vi "Master_DAQ_convertUnits.vi"(1 "Raw data in":T1={"cRIO Data"={"Time (ms)"=0.0, "24V Battery (V)"=0.0, "LowV Current (A)"=0.0, "Fiducial Sensor (V)"=0.0, "PV Pressure (psig)"=0.0, "Flow Sensor (V)"=0.0, "Temp Fairing (F)"=0.0, "Temp Reservoir (F)"=0.0, "HallEffect Right (in)"=0.0, "HallEffect Left (in)"=0.0, "PT Tank (psig)"=0.0, "PT Clamp Right (psig)"=0.0, "PT Clamp Left (psig)"=0.0, "PT Brake (psig)"=0.0, "PT Cooling (psig)"=0.0, "Displacement (ft)"=0.0, "Velocity (ft/s)"=0.0}, "IMU Data"={"x acceleration (g)"=0.0, "Pressure (psia)"=0.0, "Temperature (F)"=0.0}, "BMS Data"={"Max Cell Voltage (V)"=0.0, "Max Cell ID"=0.0, "Min Cell Voltage (V)"=0.0, "Min Cell ID"=0.0, "State of Charge (%)"=0.0, "Average Voltage (V)"=0.0, "Voltage Delta (V)"=0.0, "Pack Current (A)"=0.0, "Pack Voltage (V)"=0.0, "Max Resistance (Ohm)"=0.0, "Min Resistance (Ohm)"=0.0, "Average Resistance (Ohm)"=0.0, "Delta Resistance (Ohm)"=0.0, "Highest Temperature(F)"=0.0, "BmsStatus"={"isFault"=FALSE, "isolationMonitoring"=FALSE}}, "Motor Data"={"Velo (RPM)"=0.0, "MotorTemp(F)"=0.0, "CtrlTemp(F)"=0.0, "DcLinkVolt(V)"=0.0, "ErrorCode"=0.0, "motorStatus"={"isReady"=FALSE, "isOn"=FALSE, "isOperEn"=FALSE, "isFault"=FALSE, "isVoltEn"=FALSE, "targetReached"=FALSE, "isWarning"=FALSE}, "isAlive"=FALSE, "motorControllerState"=1}} {"Motor Data"."motorControllerState" items=["unknown"=1, "boot-up"=0, "stopped"=4, "operational"=5, "pre-operational"=127, "connection lost"=128]}) -> (0 "Data out":T1={"cRIO Data"={"Time (ms)"=0.0, "24V Battery (V)"=0.0, "LowV Current (A)"=0.0, "Fiducial Sensor (V)"=0.0, "PV Pressure (psig)"=0.0, "Flow Sensor (V)"=0.0, "Temp Fairing (F)"=0.0, "Temp Reservoir (F)"=0.0, "HallEffect Right (in)"=0.0, "HallEffect Left (in)"=0.0, "PT Tank (psig)"=0.0, "PT Clamp Right (psig)"=0.0, "PT Clamp Left (psig)"=0.0, "PT Brake (psig)"=0.0, "PT Cooling (psig)"=0.0, "Displacement (ft)"=0.0, "Velocity (ft/s)"=0.0}, "IMU Data"={"x acceleration (g)"=0.0, "Pressure (psia)"=0.0, "Temperature (F)"=0.0}, "BMS Data"={"Max Cell Voltage (V)"=0.0, "Max Cell ID"=0.0, "Min Cell Voltage (V)"=0.0, "Min Cell ID"=0.0, "State of Charge (%)"=0.0, "Average Voltage (V)"=0.0, "Voltage Delta (V)"=0.0, "Pack Current (A)"=0.0, "Pack Voltage (V)"=0.0, "Max Resistance (Ohm)"=0.0, "Min Resistance (Ohm)"=0.0, "Average Resistance (Ohm)"=0.0, "Delta Resistance (Ohm)"=0.0, "Highest Temperature(F)"=0.0, "BmsStatus"={"isFault"=FALSE, "isolationMonitoring"=FALSE}}, "Motor Data"={"Velo (RPM)"=0.0, "MotorTemp(F)"=0.0, "CtrlTemp(F)"=0.0, "DcLinkVolt(V)"=0.0, "ErrorCode"=0.0, "motorStatus"={"isReady"=FALSE, "isOn"=FALSE, "isOperEn"=FALSE, "isFault"=FALSE, "isVoltEn"=FALSE, "targetReached"=FALSE, "isWarning"=FALSE}, "isAlive"=FALSE, "motorControllerState"=1}} {"Motor Data"."motorControllerState" items=["unknown"=1, "boot-up"=0, "stopped"=4, "operational"=5, "pre-operational"=127, "connection lost"=128]})   [LabVIEW 2017]
uses:
  Master_DataControl.ctl
  TypeDef_cRIOData.ctl
  IMU/TypeDef_IMUData.ctl
  CAN/TypeDef_BMSData.ctl
  CAN/TypeDef_BMS_Status.ctl
  CAN/MotorController/fixedMotorData.ctl
  CAN/MotorController/MotorStatus.ctl
  CAN/MotorController/MotorData.ctl
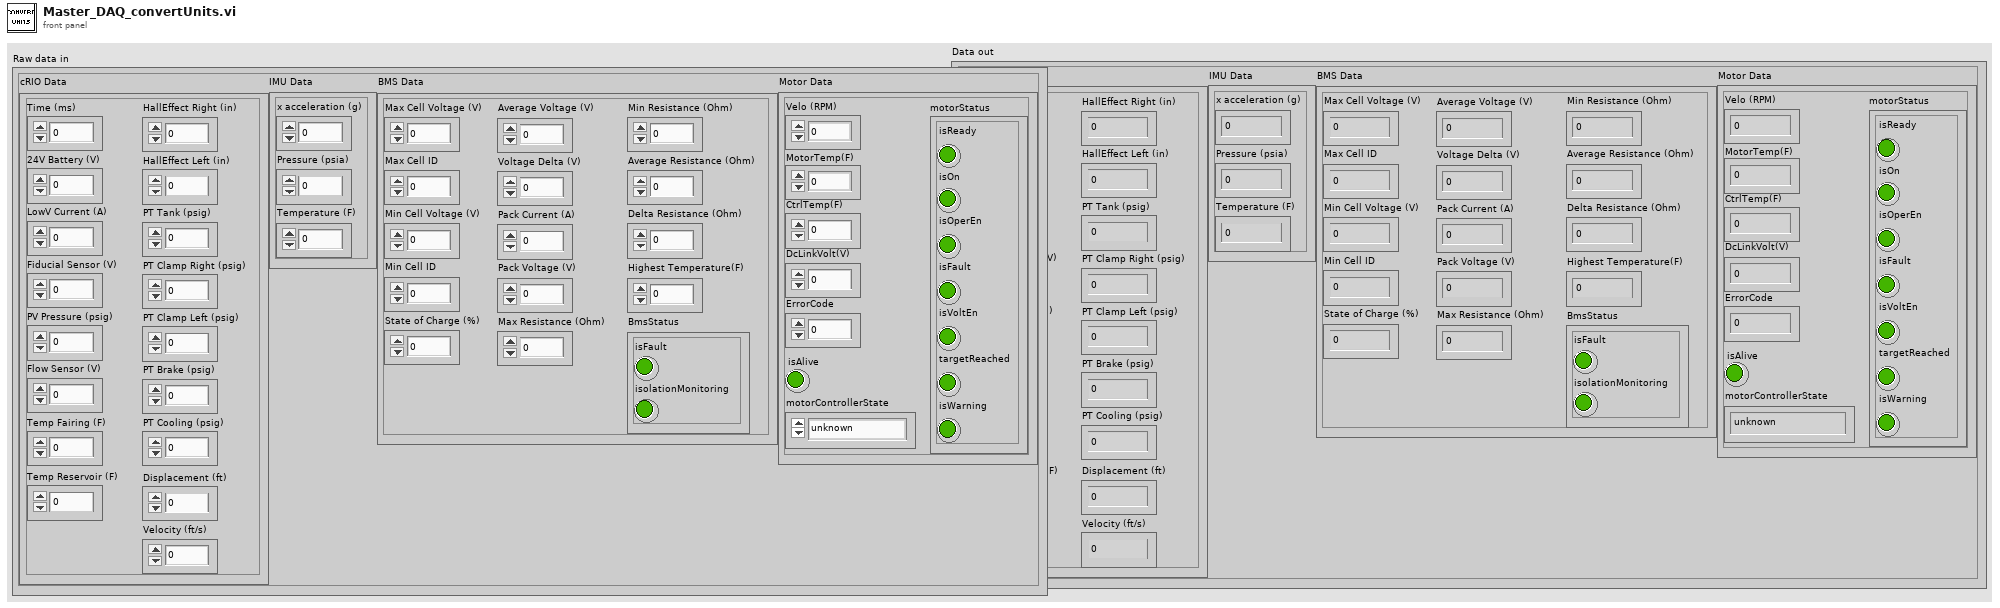
[diagram p1: front panel]
types:
  T1 = typedef "Master_DataControl.ctl" = cluster{"cRIO Data":T2, "IMU Data":T3, "BMS Data":T4, "Motor Data":T6}
  T2 = typedef "TypeDef_cRIOData.ctl" = cluster{"Time (ms)":dbl, "24V Battery (V)":dbl, "LowV Current (A)":dbl, "Fiducial Sensor (V)":dbl, "PV Pressure (psig)":dbl, "Flow Sensor (V)":dbl, "Temp Fairing (F)":dbl, "Temp Reservoir (F)":dbl, "HallEffect Right (in)":dbl, "HallEffect Left (in)":dbl, "PT Tank (psig)":dbl, "PT Clamp Right (psig)":dbl, "PT Clamp Left (psig)":dbl, "PT Brake (psig)":dbl, "PT Cooling (psig)":dbl, "Displacement (ft)":dbl, "Velocity (ft/s)":dbl}
  T3 = typedef "TypeDef_IMUData.ctl" = cluster{"x acceleration (g)":dbl, "Pressure (psia)":dbl, "Temperature (F)":dbl}
  T4 = typedef "TypeDef_BMSData.ctl" = cluster{"Max Cell Voltage (V)":dbl, "Max Cell ID":dbl, "Min Cell Voltage (V)":dbl, "Min Cell ID":dbl, "State of Charge (%)":dbl, "Average Voltage (V)":dbl, "Voltage Delta (V)":dbl, "Pack Current (A)":dbl, "Pack Voltage (V)":dbl, "Max Resistance (Ohm)":dbl, "Min Resistance (Ohm)":dbl, "Average Resistance (Ohm)":dbl, "Delta Resistance (Ohm)":dbl, "Highest Temperature(F)":dbl, "BmsStatus":T5}
  T5 = typedef "TypeDef_BMS_Status.ctl" = cluster{"isFault":bool, "isolationMonitoring":bool}
  T6 = typedef "fixedMotorData.ctl" = cluster{"Velo (RPM)":dbl, "MotorTemp(F)":dbl, "CtrlTemp(F)":dbl, "DcLinkVolt(V)":dbl, "ErrorCode":dbl, "motorStatus":T7, "isAlive":bool, "motorControllerState":u16}
  T7 = typedef "MotorStatus.ctl" = cluster{"isReady":bool, "isOn":bool, "isOperEn":bool, "isFault":bool, "isVoltEn":bool, "targetReached":bool, "isWarning":bool}
  T8 = typedef "MotorData.ctl" = cluster{"Velo (RPM)":i32, "MotorTemp(C)":u8, "CtrlTemp(C)":u8, "DcLinkVolt(V)":dbl, "ErrorCode":dbl, "isAlive":bool, "motorControllerState":u16, "motorStatus":T7}
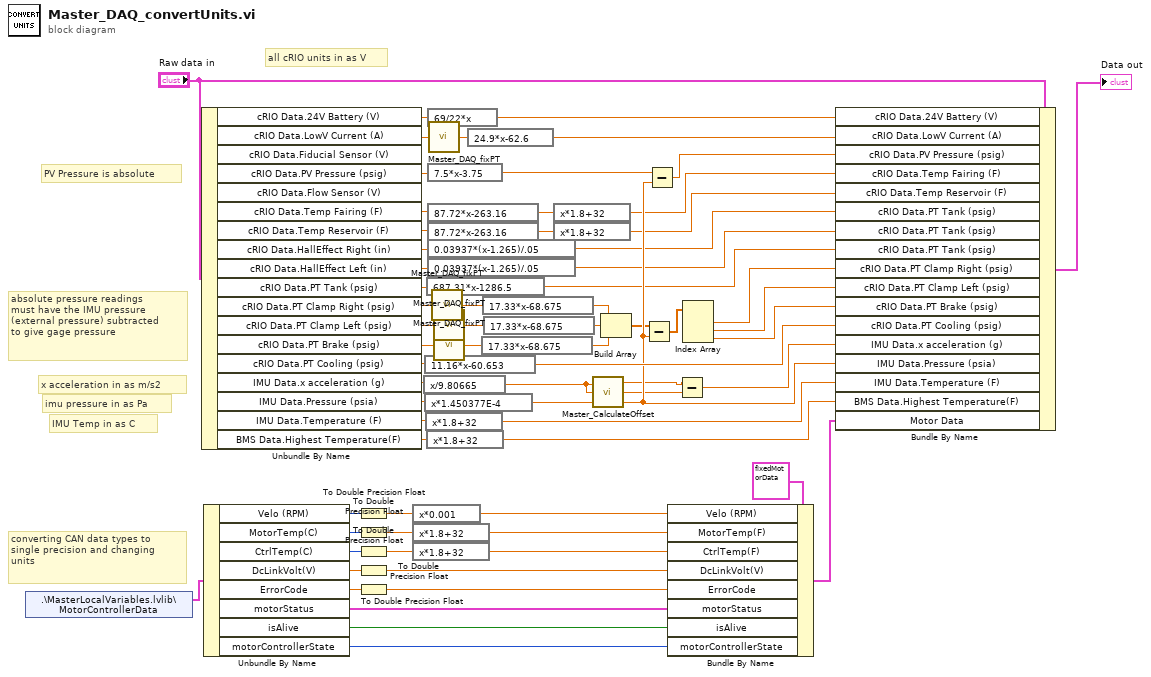
[diagram p0: block diagram]
diagram:
  # "converting CAN data types to\nsingle precision and changing\nunits"
  # "absolute pressure readings\nmust have the IMU pressure\n(external pressure) subtracted\nto give gage pressure"
  # "PV Pressure is absolute"
  # "IMU Temp in as C"
  # "imu pressure in as Pa"
  # "x acceleration in as m/s2"
  # "all cRIO units in as V"
  n1 = shared-variable ".\\MasterLocalVariables.lvlib\\MotorControllerData"() -> (w38:T8)  [unwired: 1 in, 1 out]
  n2 = Unbundle By Name("Raw data in") -> ("cRIO Data.24V Battery (V)"=w65:dbl, "cRIO Data.LowV Current (A)"=w3:dbl, "cRIO Data.PV Pressure (psig)"=w64:dbl, "cRIO Data.Temp Fairing (F)"=w63:dbl, "cRIO Data.Temp Reservoir (F)"=w62:dbl, "cRIO Data.HallEffect Right (in)"=w17:dbl, "cRIO Data.HallEffect Left (in)"=w16:dbl, "cRIO Data.PT Tank (psig)"=w61:dbl, "cRIO Data.PT Clamp Right (psig)"=w12:dbl, "cRIO Data.PT Clamp Left (psig)"=w11:dbl, "cRIO Data.PT Brake (psig)"=w10:dbl, "cRIO Data.PT Cooling (psig)"=w60:dbl, "IMU Data.x acceleration (g)"=w59:dbl, "IMU Data.Pressure (psia)"=w58:dbl, "IMU Data.Temperature (F)"=w57:dbl, "BMS Data.Highest Temperature(F)"=w56:dbl)  [unwired: 2 out]
  n3 = Unbundle By Name(w38) -> ("Velo (RPM)"=w37:i32, "MotorTemp(C)"=w35:u8, "CtrlTemp(C)"=w34:u8, "DcLinkVolt(V)"=w33:dbl, "ErrorCode"=w32:dbl, "motorStatus"=w30:T7, "isAlive"=w31:bool, "motorControllerState"=w20:u16)
  n4 = To Double Precision Float(number=w37) -> (double precision float=w29:dbl)
  n5 = To Double Precision Float(number=w35) -> (double precision float=w23:dbl)
  n6 = To Double Precision Float(number=w34) -> (double precision float=w27:dbl)
  n7 = To Double Precision Float(number=w33) -> (double precision float=w25:dbl)
  n8 = To Double Precision Float(number=w32) -> (double precision float=w26:dbl)
  n9 = expression code="x*0.001"(w29) -> (w28:dbl)
  n10 = expression code="x*1.8+32"(w23) -> (w22:dbl)
  n11 = expression code="x*1.8+32"(w27) -> (w24:dbl)
  n12 = expression code="x/9.80665"(w59) -> (w41:dbl)
  n13 = expression code="11.16*x-60.653"(w60) -> (w52:dbl)
  n14 = expression code="x*1.450377E-4"(w58) -> (w46:dbl)
  n15 = expression code="x*1.8+32"(w57) -> (w53:dbl)
  n16 = expression code="687.31*x-1286.5"(w61) -> (w15:dbl)
  n17 = expression code="x*1.8+32"(w56) -> (w54:dbl)
  n18 = expression code="69/22*x"(w65) -> (w55:dbl)
  n19 = expression code="7.5*x-3.75"(w64) -> (w48:dbl)
  n20 = expression code="87.72*x-263.16"(w63) -> (w44:dbl)
  n21 = expression code="87.72*x-263.16"(w62) -> (w45:dbl)
  n22 = expression code="0.03937*(x-1.265)/.05"(w17) -> (w13:dbl)
  n23 = expression code="0.03937*(x-1.265)/.05"(w16) -> (w14:dbl)
  n24 = call "Master_DAQ_fixPT.vi"("new value"=w3) -> ("mean"=w2:dbl)
  n25 = call "Master_DAQ_fixPT.vi"("new value"=w12) -> ("mean"=w9:dbl)
  n26 = call "Master_DAQ_fixPT.vi"("new value"=w11) -> ("mean"=w8:dbl)
  n27 = call "Master_DAQ_fixPT.vi"("new value"=w10) -> ("mean"=w7:dbl)
  n28 = expression code="24.9*x-62.6"(w2) -> (w1:dbl)
  n29 = expression code="17.33*x-68.675"(w7) -> (w6:dbl)
  n30 = expression code="17.33*x-68.675"(w9) -> (w4:dbl)
  n31 = expression code="17.33*x-68.675"(w8) -> (w5:dbl)
  n32 = expression code="x*1.8+32"(w44) -> (w43:dbl)
  n33 = expression code="x*1.8+32"(w45) -> (w42:dbl)
  n34 = call "Master_CalculateOffset.vi"("Acceleration"=w41) -> ("Offset"=w40:dbl)
  n35 = Build Array(w4, w5, w6) -> (w19:dbl[])
  n36 = Subtract(x=w19, y=w46) -> (x-y=w18:dbl[])
  n37 = Subtract(x=w48, y=w46) -> (x-y=w47:dbl)
  n38 = Bundle By Name(cluster=T6 {"Velo (RPM)"=0.0, "MotorTemp(F)"=0.0, "CtrlTemp(F)"=0.0, "DcLinkVolt(V)"=0.0, "ErrorCode"=0.0, "motorStatus"={"isReady"=FALSE, "isOn"=FALSE, "isOperEn"=FALSE, "isFault"=FALSE, "isVoltEn"=FALSE, "targetReached"=FALSE, "isWarning"=FALSE}, "isAlive"=FALSE, "motorControllerState"=1} ("motorData"), "Velo (RPM)"=w28, "MotorTemp(F)"=w22, "CtrlTemp(F)"=w24, "DcLinkVolt(V)"=w25, "ErrorCode"=w26, "motorStatus"=w30, "isAlive"=w31, "motorControllerState"=w20) -> (w21:T6)
  n39 = Subtract(x=w41, y=w40) -> (x-y=w39:dbl)
  n40 = Index Array(array=w18) -> (element #1=w51:dbl, element #2=w50:dbl, element #3=w49:dbl)  [unwired: 3 in]
  n41 = Bundle By Name(cluster="Raw data in", "cRIO Data.24V Battery (V)"=w55, "cRIO Data.LowV Current (A)"=w1, "cRIO Data.PV Pressure (psig)"=w47, "cRIO Data.Temp Fairing (F)"=w43, "cRIO Data.Temp Reservoir (F)"=w42, "cRIO Data.PT Tank (psig)"=w13, "cRIO Data.PT Tank (psig)"=w14, "cRIO Data.PT Tank (psig)"=w15, "cRIO Data.PT Clamp Right (psig)"=w51, "cRIO Data.PT Clamp Left (psig)"=w50, "cRIO Data.PT Brake (psig)"=w49, "cRIO Data.PT Cooling (psig)"=w52, "IMU Data.x acceleration (g)"=w39, "IMU Data.Pressure (psia)"=w46, "IMU Data.Temperature (F)"=w53, "BMS Data.Highest Temperature(F)"=w54, "Motor Data"=w21) -> (→"Data out":T1)
